vi "ResetSprites.vi"(8 "error in (no error)":errorcluster, 11 "Game in":refnum<class "Game.lvclass">) -> (0 "error out":errorcluster, 3 "Game out":refnum<class "Game.lvclass">)   [LabVIEW 2019, in "RT_Game.lvlib" / "Game.lvclass"]
uses:
  Game.lvclass
  FPGA/Sprite/SpriteData.ctl
  Game.lvclass/Game.ctl
  <vilib>/Utility/error.llb/Error Cluster From Error Code.vi
  <vilib>/rvi/errors/niLvFpgaAdjustHostInterfaceError.vi
  <vilib>/rvi/interface/nirviReadWriteControl/nirviReadWriteControl.xnode
  FPGA_Interface.ctl
  FPGA Bitfiles/myriogameconsole_FPGATarget_Main_ntsPRcBZGxk.lvbitx
  FPGA/Sprite/Sprite.lvlib
  NiFpgaLv.dll
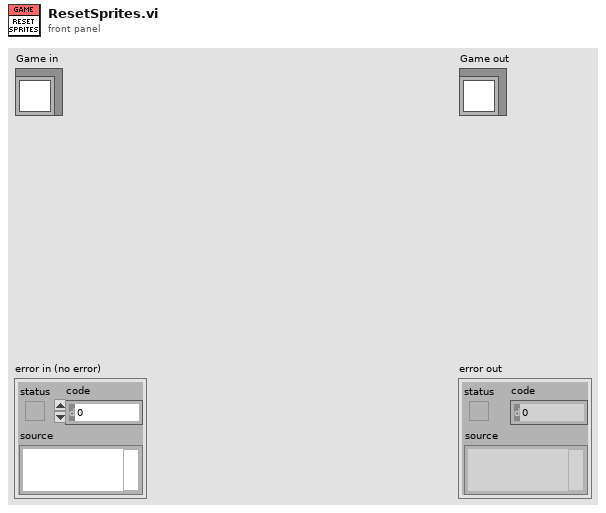
[diagram p1: front panel]
types:
  T1 = typedef "Sprite.lvlib/SpriteData.ctl" = cluster{"Pos_X":i16, "Pos_Y":i16, "Width":i16, "Height":i16, "BufferIndex":i16, "TransparencyColor":fxp<+,3,3>}
  T2 = typedef "FPGA_Interface.ctl" = refnum<k20>
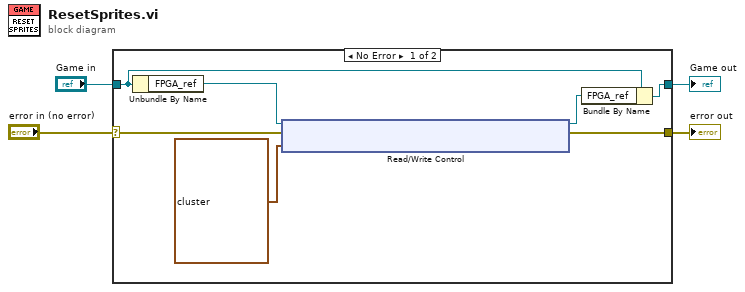
[diagram p0: block diagram]
diagram:
  n1 = case shown="No Error" "error in (no error)" {
    selector: "error in (no error)" -> [w11 w13]
    tunnel: [w8 w13] -> w3
    tunnel: [w9 w12] -> w1
    tunnel: "Game in" -> [w10 w12]
    frame No Error {
      n2 = Unbundle By Name(w10) -> ("FPGA_ref"=w7:T2)
      n3 = xnode "Read/Write Control"("FPGA VI Reference In"=w7, "error in"=w11, "Sprites"=T1[] [{"Pos_X"=0, "Pos_Y"=0, "Width"=0, "Height"=0, "BufferIndex"=0, "TransparencyColor"=0.0}, {"Pos_X"=0, "Pos_Y"=0, "Width"=0, "Height"=0, "BufferIndex"=0, "TransparencyColor"=0.0}, {"Pos_X"=0, "Pos_Y"=0, "Width"=0, "Height"=0, "BufferIndex"=0, "TransparencyColor"=0.0}]) -> ("FPGA VI Reference Out"=w6:T2, "error out"=w8:errorcluster)
      n4 = Bundle By Name(cluster=w10, "FPGA_ref"=w6) -> (w9:refnum<class "Game.lvclass">)
    }
    frame Error {
    }
  }
  "error out" <- w3
  "Game out" <- w1
